vi "Copy New Source To Install.vi"(8 "Error In":errorcluster, 9 "Install Root":string, 10 "Source Root":string, 11 "All Files Source Files":path[](array[path])) -> (0 "Error Out":errorcluster, 1 "Install Root":string, 2 "Source Root":string)   [LabVIEW 2011, in "LVH-Build-Tools.lvlib"]
doc: "This VI copies files from the source directory to the appropriate directory under the install root and replaces the source file with a hard link to the installed file. The user is prompted to overwrite if the file already exists."
uses:
  LVH-Build-Tools.lvlib
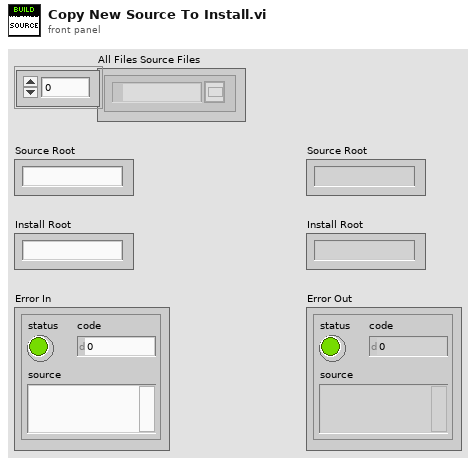
[diagram p1: front panel]
types:
  T1 = typedef "LVH-Build-Tools.lvlib/Configuration.ctl" = cluster{"Source Root":string, "Install Root":string, "Components":string[], "Ignore":string[]}
  T2 = enum16{"Left Button", "Center Button", "Right Button", "Window Close"}
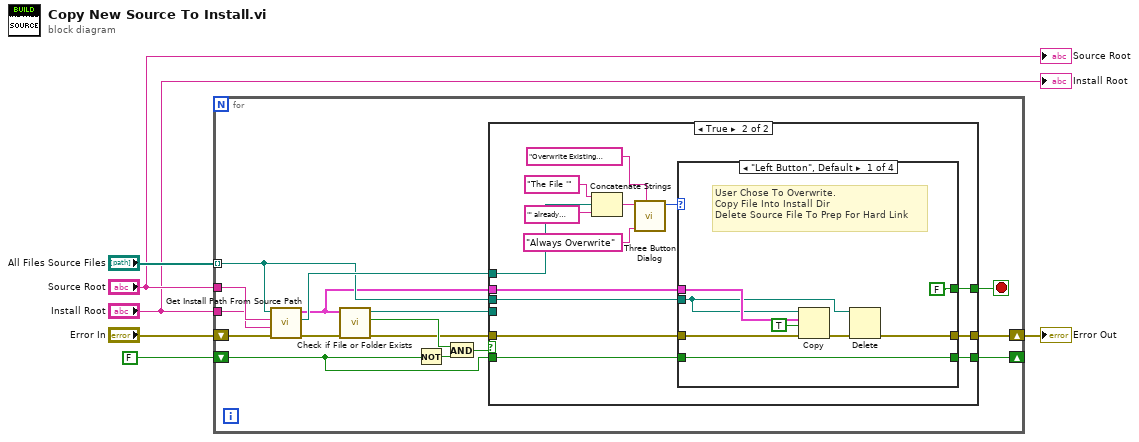
[diagram p0: block diagram]
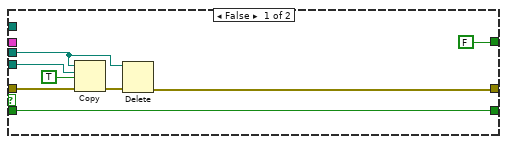
[diagram p2: hidden frame]
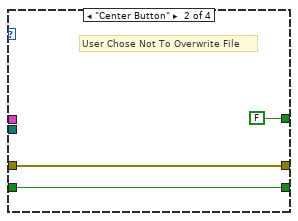
[diagram p3: hidden frame]
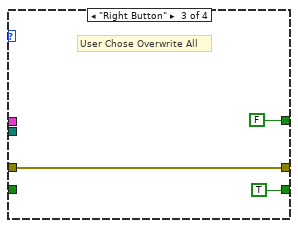
[diagram p4: hidden frame]
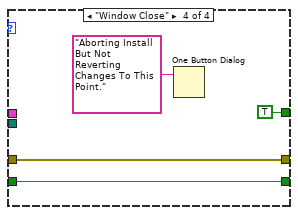
[diagram p5: hidden frame]
diagram:
  n1 = for {
    tunnel: "All Files Source Files" -> [w12] mode=indexing
    tunnel: "Source Root" -> [w21]
    tunnel: "Install Root" -> [w20]
    shift-right: [w8] -> _
    shift-left: FALSE ("overwrite (F)") -> [w13]
    shift-right: [w9] -> w1
    shift-left: "Error In" -> [w22]
    stop <- w7 stop-if-true
    n2 = call "Get Install Path From Source Path.vi"("Error In"=w22, 9:w20, "Source File Path"=w21, "Configuration"=w12) -> ("Error Out"=w19:errorcluster, "Install File Path"=w17:path, "Configuration"=w11:T1)  [unwired: 4 in, 1 out]
    n3 = call <vilib>:"Check if File or Folder Exists.vi"("error in (no error)"=w19, "path"=w11) -> ("error out"=w10:errorcluster, "file or folder exists?"=w14:bool, "dup path"=w18:path)  [unwired: 7 in]
    n4 = Not(x=w13) -> (.not. x?=w16:bool)
    n5 = And(x=w14, y=w16) -> (x .and. y?=w15:bool)
    n6 = case shown="True" w15 {
      tunnel: w18 -> [w30 _]
      tunnel: w17 -> [_ w43]
      tunnel: w13 -> [w27 w32]
      tunnel: w12 -> [w24 w37]
      tunnel: w11 -> [_ w36]
      tunnel: w10 -> [w28 w35]
      tunnel: [w23 w34] -> w9
      tunnel: [w27 w33] -> w8
      tunnel: [FALSE w31] -> w7
      frame False {
        n7 = Copy(8:w28, 9:TRUE ("overwrite (F)"), 10:w30, 11:w24) -> (0:w25:errorcluster)  [unwired: 1 in, 2 out]
        n8 = Delete(path (use dialog)=w24, error in=w25) -> (error out=w23:errorcluster)  [unwired: 3 in, 2 out]
      }
      frame True {
        n9 = Concatenate Strings("The File '" ("string"), w43, "' already exists in the install directory.  Do you want to overwrite it?" ("string")) -> (w41:string)
        n10 = call <vilib>:"Three Button Dialog.vi"("Window Title (\"\")"="Overwrite Existing Installed File?" ("Window Title (\"\")"), "Right Button Text (\"Cancel\")"="Always Overwrite" ("Right Button Text (\"Cancel\")"), "message"=w41) -> ("Which Button?"=w38:T2)  [unwired: 8 in]
        n11 = case shown="\"Left Button\", Default" w38 {
          tunnel: w37 -> [w45 _ _ _]
          tunnel: w36 -> [w52 _ _ _]
          tunnel: w35 -> [w50 w55 w56 w60]
          tunnel: [w46 w55 w56 w60] -> w34
          tunnel: [w49 w54 TRUE ("overwrite (F)") w62] -> w33
          tunnel: w32 -> [w49 w54 _ w62]
          tunnel: [FALSE FALSE FALSE TRUE] -> w31
          frame "Left Button", Default {
            # "User Chose To Overwrite.\nCopy File Into Install Dir\nDelete Source File To Prep For Hard Link"
            n12 = Copy(8:w50, 9:TRUE ("overwrite (F)"), 10:w52, 11:w45) -> (0:w47:errorcluster)  [unwired: 1 in, 2 out]
            n13 = Delete(path (use dialog)=w45, error in=w47) -> (error out=w46:errorcluster)  [unwired: 3 in, 2 out]
          }
          frame "Center Button" {
            # "User Chose Not To Overwrite File"
          }
          frame "Right Button" {
            # "User Chose Overwrite All"
          }
          frame "Window Close" {
            n14 = One Button Dialog(message="Aborting Install But Not Reverting Changes To This Point.") -> ()  [unwired: 1 in, 1 out]
          }
        }
      }
    }
  }
  "Error Out" <- w1
  "Source Root" <- "Source Root"
  "Install Root" <- "Install Root"
